vi "replace by name.vi"(8 "error in (no error)":errorcluster, 10 "New object":refnum<class "system object.lvclass">, 11 "SysObj in":refnum<class "Folder.lvclass">) -> (0 "error out":errorcluster, 1 "Replaced":bool, 3 "SysObj out":refnum<class "system object.lvclass">)   [LabVIEW 2020, in "Folder.lvclass"]
uses:
  Folder.lvclass
  C:/PA_Source/advent-of-code/2022/Paul/07/classes/system object/system object.lvclass
  system object/system object.lvclass
  Folder.lvclass/Folder.ctl
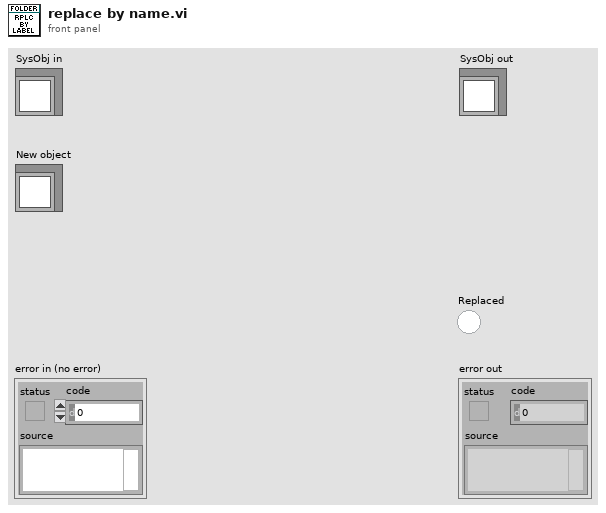
[diagram p1: front panel]
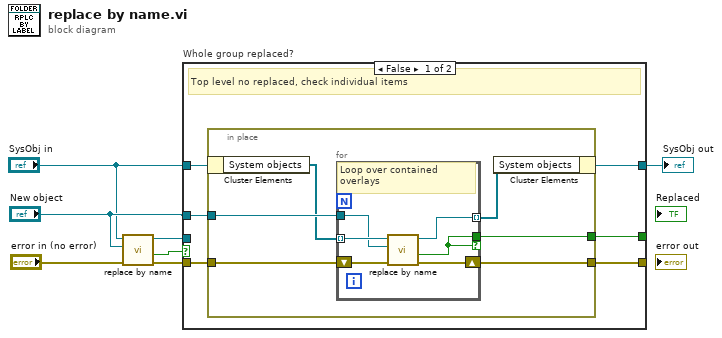
[diagram p0: block diagram]
diagram:
  n1 = call-parent "replace by name.vi"("error in (no error)"="error in (no error)", "New object"="New object", "SysObj in"="SysObj in") -> ("error out"=w6:errorcluster, "Replaced"=w5:bool, "SysObj out"=w4:refnum<class "system object.lvclass">)  [unwired: 6 in]
  n2 = case "Whole group replaced?" shown="False" w5 {
    selector: w5 -> [_ w27]
    tunnel: [w8 w28] -> w1
    tunnel: w4 -> [_ w28]
    tunnel: [w12 w27] -> _
    tunnel: "SysObj in" -> [w9 _]
    tunnel: "New object" -> [w13 _]
    tunnel: w6 -> [w11 w26]
    tunnel: [w10 w26] -> _
    frame False {
      # "Top level no replaced, check individual items"
      n3 = in-place {
        in-place-border: w13 -> [w19]
        in-place-border: [w18] -> w12
        in-place-border: w11 -> [w17]
        in-place-border: [w16] -> w10
        n4 = in-place-cluster #1(w9) -> ("System objects"=w15:refnum<class "system object.lvclass">[])
        n5 = for {
          tunnel: w15 -> [w23] mode=indexing
          tunnel: w19 -> [w22]
          tunnel: [w21] -> w14 mode=indexing
          tunnel: [w20] -> w18 if=w20
          shift-right: [w24] -> w16
          shift-left: w17 -> [w25]
          # "Loop over contained overlays"
          n6 = call-dynamic "replace by name.vi"("error in (no error)"=w25, "New object"=w22, "SysObj in"=w23) -> ("error out"=w24:errorcluster, "Replaced"=w20:bool, "SysObj out"=w21:refnum<class "system object.lvclass">)  [unwired: 6 in]
        }
        n7 = in-place-cluster #1("System objects"=w14) -> (w8:refnum<class "Folder.lvclass">)
      }
    }
    frame True {
      # "Whole group replaced - return new overlay"
    }
  }
  "SysObj out" <- w1
